vi "LVDemo1.vi"() -> ()   [LabVIEW 2010]
uses:
  toupcam.dll
  toupcam_labview.dll
panel:
  in  "Temp 3":i32
  in  "Tint 3":i32
  in  "Expotime 3":u32
  in  "ExpoGain 3":u16
  in  "Still_Width 2":i32
  in  "Still_Height 2":i32
  in  "Tab":T1(tab)
  in  "Color Default":bool
  in  "Brightness":i32(slide) scale=-64.0..64.0
  in  "Contrast":i32(slide) scale=-100.0..100.0
  in  "Gamma":i32(slide) scale=20.0..180.0
  in  "Hue":i32(slide) scale=-180.0..180.0
  in  "Saturation":i32(slide) scale=0.0..255.0
  in  "AutoExpo":bool
  in  "ExpoDefault":bool
  in  "Expotime":u32(slide) scale=294.0..2000000.0
  in  "ExpoGain":u16(slide) scale=100.0..300.0
  in  "AutoWB":bool
  in  "WBDefault":bool
  in  "Tint":i32(slide) scale=200.0..2500.0
  in  "Temp":i32(slide) scale=2000.0..15000.0
  in  "Bin/Skip Mode":bool
  in  "Chrome/Mono":bool
  in  "HFlip":bool
  in  "VFlip":bool
  in  "Frame Speed":u8(slide) scale=0.0..6.0
  out "Video":T2(plugin-control)
  in  "Cap Still Image":bool
  in  "Still Image Resolution":u16(ring) items=["2592*1944", "1280*960", "640*480"]
  in  "Cap Live Image":bool
  in  "Stop":bool
  in  "Live Resolution":u16(ring) items=["2592*1944", "1280*960", "640*480"]
  in  "?":enum32{"选项卡 1"}(tab)
  in  "Expotime_def":u32
  in  "ExpoGain_def":u16
  in  "ExpoGain_Max":u16
  in  "ExpoGain_Min":u16
  in  "Height":i32
  in  "Width":i32
  in  "Expotime_Max":u32
  in  "Expotime_Min":u32
  in  "speed":u8
  in  "height2":i32
  in  "width2":i32
  in  "Mode":bool
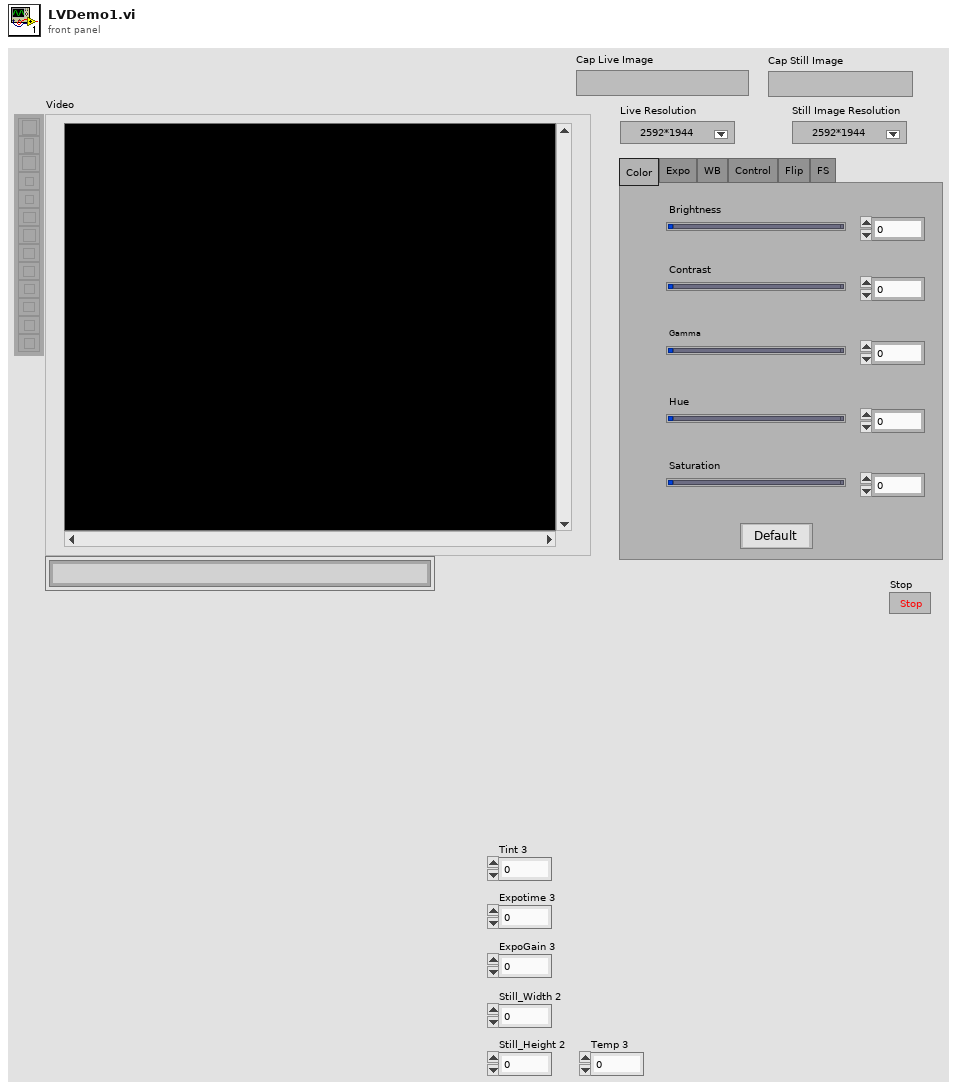
[diagram p1: front panel]
types:
  T1 = enum32{"Color", "Expo", "WB", "Control", "Flip", "FS"}
  T2 = typedef "IMAQ Image.ctl" = refnum<image>
  T3 = enum8{"Enabled", "Disabled", "Disabled and Grayed Out"}
  T4 = typedef "Image Type" = u32
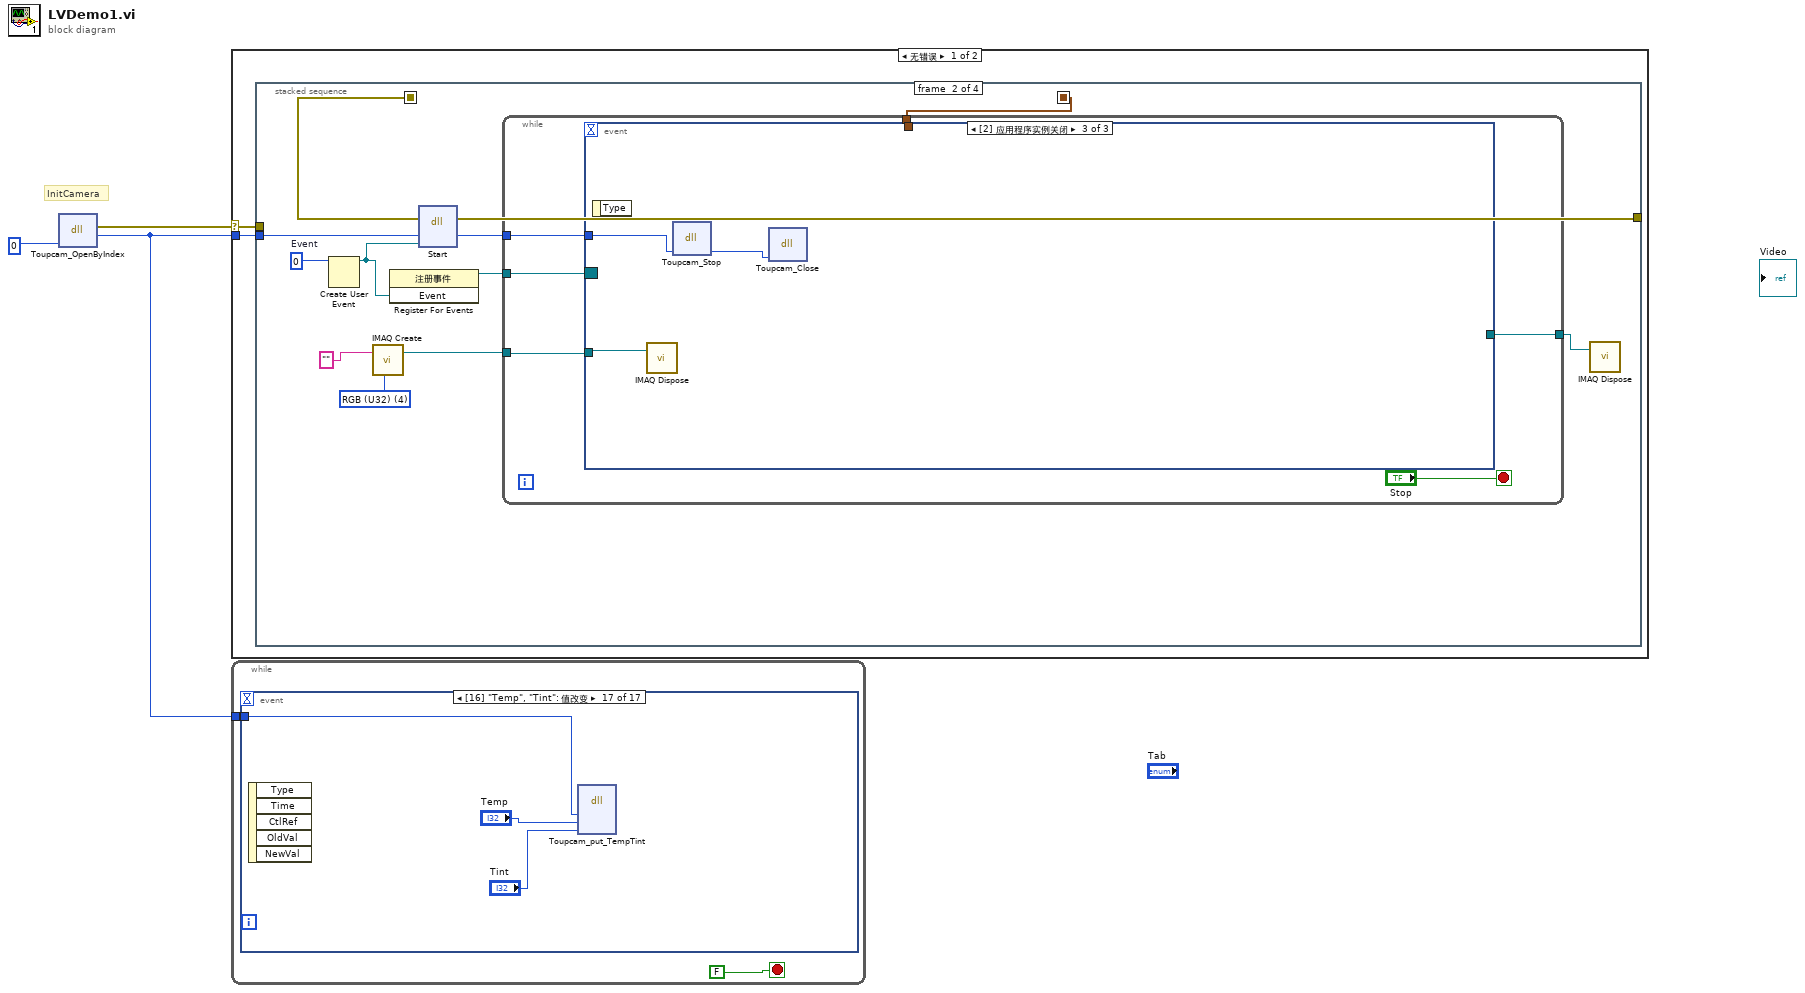
[diagram p0: block diagram]
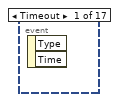
[diagram p2: hidden frame]
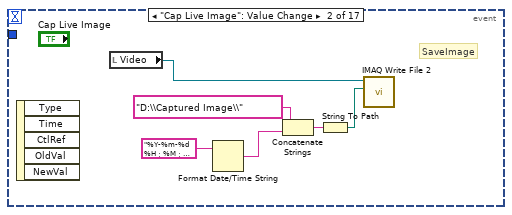
[diagram p3: hidden frame]
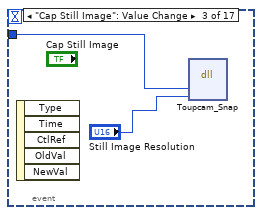
[diagram p4: hidden frame]
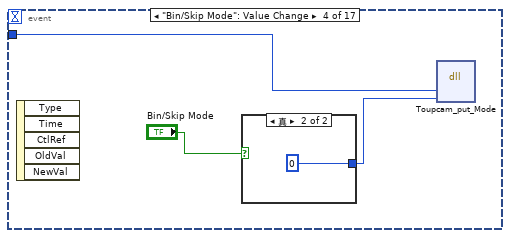
[diagram p5: hidden frame]
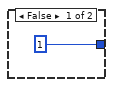
[diagram p6: hidden frame]
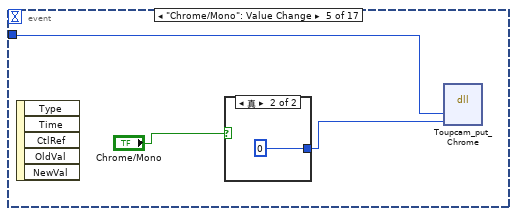
[diagram p7: hidden frame]
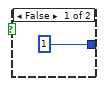
[diagram p8: hidden frame]
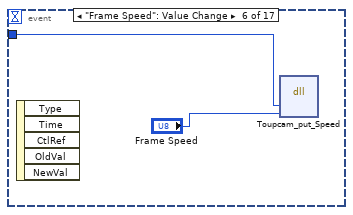
[diagram p9: hidden frame]
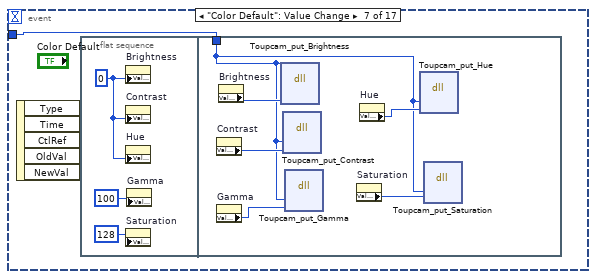
[diagram p10: hidden frame]
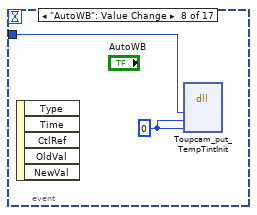
[diagram p11: hidden frame]
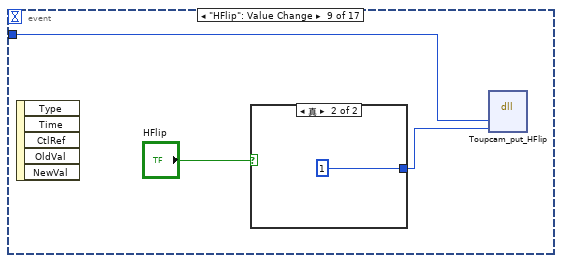
[diagram p12: hidden frame]
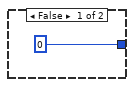
[diagram p13: hidden frame]
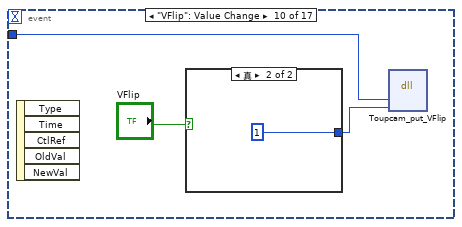
[diagram p14: hidden frame]
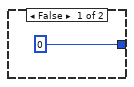
[diagram p15: hidden frame]
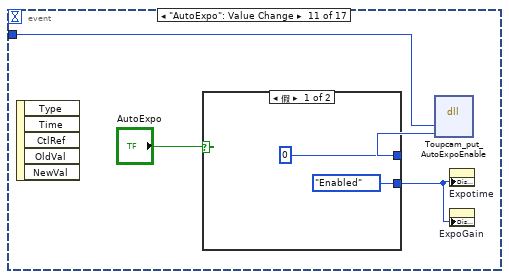
[diagram p16: hidden frame]
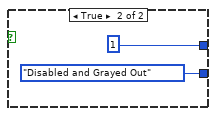
[diagram p17: hidden frame]
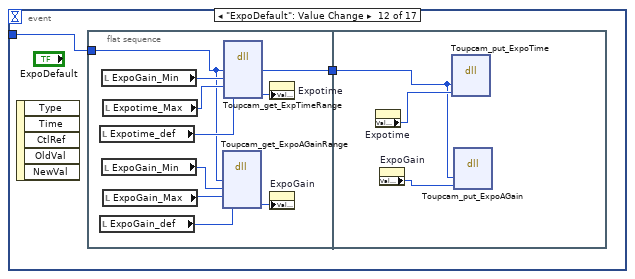
[diagram p18: hidden frame]
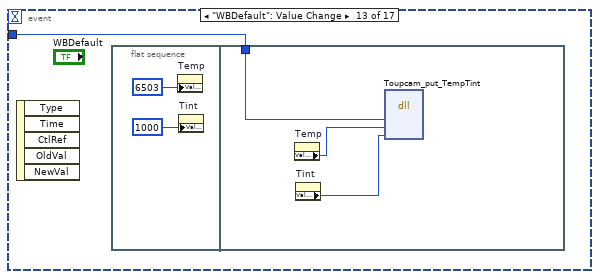
[diagram p19: hidden frame]
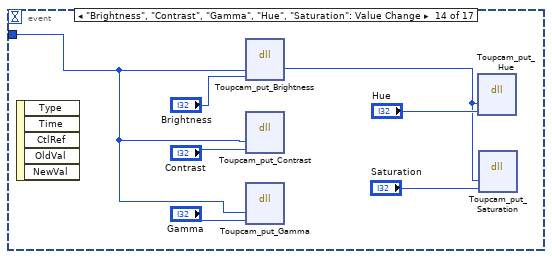
[diagram p20: hidden frame]
diagram:
  # "InitCamera"
  n1 = dll-call lib="C:/LVDemo x86/toupcam.dll" fn="Toupcam_OpenByIndex"("Index"=0) -> (error out=w3:errorcluster, "return type"=w2:i32)  [unwired: 4 in, 1 out]
  n2 = case shown="无错误" w3 {
    selector: w3 -> [w4 _]
    tunnel: w2 -> [w5 _]
    frame No Error {
      n3 = stacked-sequence {
        seq-local: [w26 _ _ _] -> [_ w72 _ _]
        seq-local: [w24 _ _ _] -> [_ w71 _ _]
        tunnel: w5 -> [w9 w69 w132 w135]
        tunnel: w4 -> [w24 _ _ w134]
        tunnel: [_ w70 _ _] -> _
        frame #0 {
          w6 = T3."Disabled and Grayed Out" ("禁用")
          w47 = 0
          # "SetSliderRange"
          # "SetCameraResolution"
          # "CameraResolution"
          # "SetSliderDefault"
          n4 = dll-call lib="C:/LVDemo x86/toupcam.dll" fn="Toupcam_put_AutoExpoEnable"("htoupcam"=w9, "bAutoExposure"=FALSE) -> ()  [unwired: 6 in, 2 out]
          n5 = dll-call lib="C:/LVDemo x86/toupcam.dll" fn="Toupcam_put_ExpoTime"("htoupcam"=w9, "Time"=5000) -> ()  [unwired: 6 in, 2 out]
          n6 = dll-call lib="C:/LVDemo x86/toupcam.dll" fn="Toupcam_get_ExpTimeRange"("htoupcam"=w9, "nMin"="Expotime_Min", "nMax"="Expotime_Max", "ndef"="Expotime_def") -> ("nMin"=w29:u32, "nMax"=w28:u32, "ndef"=w27:u32)  [unwired: 5 in, 2 out]
          n7 = dll-call lib="C:/LVDemo x86/toupcam.dll" fn="Toupcam_get_ExpoAGainRange"("htoupcam"=w9, "nmin"="ExpoGain_Min", "nmax"="ExpoGain_Max", "ndef"="ExpoGain_def") -> ("nmin"=w38:u16, "nmax"=w37:u16, "ndef"=w36:u16)  [unwired: 5 in, 2 out]
          n8 = property on="Expotime" class="Slide (strict)"("Scale.Minimum"=w29, "Scale.Maximum"=w28, "Value"=w27) -> ()  [unwired: 2 in, 2 out]
          n9 = property on="ExpoGain" class="Slide (严格)"("Scale.Minimum"=w38, "Scale.Maximum"=w37, "Value"=w36) -> ()  [unwired: 2 in, 2 out]
          n10 = dll-call lib="C:/LVDemo x86/toupcam.dll" fn="Toupcam_get_ResolutionNumber"("htoupcam"=w9) -> ("返回类型"=w15:u32, "htoupcam"=w14:i32)  [unwired: 3 in, 2 out]
          n11 = dll-call lib="C:/LVDemo x86/toupcam.dll" fn="Toupcam_get_Mode"("htoupcam"=w9, "bMode"="Mode") -> ("返回类型"=w8:i32)  [unwired: 5 in, 2 out]
          n12 = property on="Expotime" class="Slide (strict)"("DisabledEnum"=w6) -> ()  [unwired: 2 in, 2 out]
          n13 = property on="ExpoGain" class="Slide (strict)"("DisabledEnum"=w6) -> ()  [unwired: 2 in, 2 out]
          n14 = Equal To 0?(x=w8) -> (x = 0?=w7:bool)
          n15 = dll-call lib="C:/LVDemo x86/toupcam.dll" fn="Toupcam_get_MaxSpeed"("htoupcam"=w9) -> ("返回类型"=w19:u8)  [unwired: 4 in, 2 out]
          n16 = dll-call lib="C:/LVDemo x86/toupcam.dll" fn="Toupcam_get_Speed"("htoupcam"=w9, "speed"="speed") -> ("htoupcam"=w17:i32, "speed"=w20:u8)  [unwired: 4 in, 2 out]
          n17 = for {
            N: w15 -> [_]
            tunnel: w14 -> [w61]
            tunnel: [w52] -> w13 mode=indexing
            i -> [w53]
            # "Enum Res"
            n18 = dll-call lib="C:/LVDemo x86/toupcam.dll" fn="Toupcam_get_Resolution"("htoupcam"=w61, "ResNum"=w53, "pWidth"="width2", "pHeight"="height2") -> ("pWidth"=w55:i32, "pHeight"=w54:i32)  [unwired: 6 in, 2 out]
            n19 = Number To Decimal String(number=w55) -> (decimal integer string=w56:string)  [unwired: 1 in]
            n20 = Number To Decimal String(number=w54) -> (decimal integer string=w58:string)  [unwired: 1 in]
            n21 = Concatenate Strings(w56, "*", w58) -> (w52:string)
          }
          n22 = case shown="假" w7 {
            frame True {
              n23 = property on="Bin/Skip Mode" class="Bool (严格)"("DisabledEnum"=T3."Enabled" ("禁用")) -> ()  [unwired: 2 in, 2 out]
            }
            frame False {
              n24 = property on="Bin/Skip Mode" class="Bool (严格)"("DisabledEnum"=T3."Disabled and Grayed Out" ("禁用")) -> ()  [unwired: 2 in, 2 out]
            }
          }
          n25 = property on="Frame Speed" class="Slide (严格)"("Value"=w20, "Scale.Maximum"=w19, "Scale.Minimum"=0) -> ()  [unwired: 2 in, 2 out]
          n26 = dll-call lib="C:/LVDemo x86/toupcam.dll" fn="Toupcam_get_MonoMode"("htoupcam"=w17) -> ("返回类型"=w16:i32)  [unwired: 4 in, 2 out]
          n27 = case shown="0, 默认" w16 {
            frame 0, Default {
              w62 = T3."Disabled and Grayed Out" ("禁用")
              # "Mono"
              n28 = property on="Brightness" class="Slide (严格)"("DisabledEnum"=w62) -> ()  [unwired: 2 in, 2 out]
              n29 = property on="Hue" class="Slide (严格)"("DisabledEnum"=w62) -> ()  [unwired: 2 in, 2 out]
              n30 = property on="Contrast" class="Slide (严格)"("DisabledEnum"=w62) -> ()  [unwired: 2 in, 2 out]
              n31 = property on="Gamma" class="Slide (严格)"("DisabledEnum"=w62) -> ()  [unwired: 2 in, 2 out]
              n32 = property on="AutoWB" class="Bool"("DisabledEnum"=w62) -> ()  [unwired: 2 in, 2 out]
              n33 = property on="Temp" class="Slide (严格)"("DisabledEnum"=w62) -> ()  [unwired: 2 in, 2 out]
              n34 = property on="Tint" class="Slide (严格)"("DisabledEnum"=w62) -> ()  [unwired: 2 in, 2 out]
              n35 = property on="Saturation" class="Slide (严格)"("DisabledEnum"=w62) -> ()  [unwired: 2 in, 2 out]
              n36 = property on="WBDefault" class="Bool"("DisabledEnum"=w62) -> ()  [unwired: 2 in, 2 out]
              n37 = property on="Color Default" class="Bool"("DisabledEnum"=w62) -> ()  [unwired: 2 in, 2 out]
            }
            frame 1 {
              w63 = T3."Enabled" ("禁用")
              # "Mono"
              n38 = property on="Brightness" class="Slide (严格)"("DisabledEnum"=w63) -> ()  [unwired: 2 in, 2 out]
              n39 = property on="Hue" class="Slide (严格)"("DisabledEnum"=w63) -> ()  [unwired: 2 in, 2 out]
              n40 = property on="Contrast" class="Slide (严格)"("DisabledEnum"=w63) -> ()  [unwired: 2 in, 2 out]
              n41 = property on="Gamma" class="Slide (严格)"("DisabledEnum"=w63) -> ()  [unwired: 2 in, 2 out]
              n42 = property on="AutoWB" class="Bool"("DisabledEnum"=w63) -> ()  [unwired: 2 in, 2 out]
              n43 = property on="Temp" class="Slide (严格)"("DisabledEnum"=w63) -> ()  [unwired: 2 in, 2 out]
              n44 = property on="Tint" class="Slide (严格)"("DisabledEnum"=w63) -> ()  [unwired: 2 in, 2 out]
              n45 = property on="Saturation" class="Slide (严格)"("DisabledEnum"=w63) -> ()  [unwired: 2 in, 2 out]
              n46 = property on="WBDefault" class="Bool"("DisabledEnum"=w63) -> ()  [unwired: 2 in, 2 out]
              n47 = property on="Color Default" class="Bool"("DisabledEnum"=w63) -> ()  [unwired: 2 in, 2 out]
            }
          }
          n48 = dll-call lib="C:/LVDemo x86/toupcam.dll" fn="Toupcam_get_Resolution"("htoupcam"=w14, "ResNum"="Live Resolution", "pWidth"="Width", "pHeight"="Height") -> ("pWidth"=w39:i32, "pHeight"=w40:i32)  [unwired: 6 in, 2 out]
          n49 = dll-call lib="C:/LVDemo x86/toupcam.dll" fn="Toupcam_put_eSize"("htoupcam"=w14, "nResolutionIndex"="Live Resolution") -> ()  [unwired: 6 in, 2 out]
          n50 = property on="Live Resolution" class="Ring (严格)"("Strings []"=w13) -> ()  [unwired: 2 in, 2 out]
          n51 = property on="Still Image Resolution" class="Ring (严格)"("Strings []"=w13) -> ()  [unwired: 2 in, 2 out]
          n52 = Bundle("pWidth"=w39, "pHeight"=w40) -> (w26:cluster{"pWidth":i32, "pHeight":i32})  [unwired: 1 in]
          n53 = property on="Brightness" class="Slide (严格)"("Value"=w47) -> ()  [unwired: 2 in, 2 out]
          n54 = property on="Contrast" class="Slide (严格)"("Value"=w47) -> ()  [unwired: 2 in, 2 out]
          n55 = property on="Hue" class="Slide (严格)"("Value"=w47) -> ()  [unwired: 2 in, 2 out]
          n56 = property on="Gamma" class="Slide (严格)"("Value"=100) -> ()  [unwired: 2 in, 2 out]
          n57 = property on="Saturation" class="Slide (严格)"("Value"=128) -> ()  [unwired: 2 in, 2 out]
          n58 = property on="Temp" class="Slide (严格)"("Value"=6503) -> ()  [unwired: 2 in, 2 out]
          n59 = property on="Tint" class="Slide (严格)"("Value"=1000) -> ()  [unwired: 2 in, 2 out]
          n60 = property on="AutoExpo" class="Bool (严格)"("Value"=TRUE) -> ()  [unwired: 2 in, 2 out]
          n61 = property on="Bin/Skip Mode" class="Bool (严格)"("Value"=TRUE) -> ()  [unwired: 2 in, 2 out]
          n62 = property on="Chrome/Mono" class="Bool (严格)"("Value"=TRUE) -> ()  [unwired: 2 in, 2 out]
          n63 = property class="TabCtl (严格)"("Visible"=FALSE) -> ()  [unwired: 2 in, 2 out]
        }
        frame #1 {
          w68 = u32 0  # Event
          w73 = T4 4 items=["Grayscale (U8)", "Grayscale (I16)", "Grayscale (SGL)", "Complex (CSG)", "RGB (U32)", "HSL (U32)", "RGB (U64)", "Grayscale (U16)"] ("Image Type")
          n64 = Create User Event(user event datatype=w68) -> (user event=w67:refnum<user-event>)  [unwired: 1 in, 1 out]
          n65 = call "IMAQ Create"("Image Name"="", "Image Type"=w73) -> ("New Image"=w74:T2)  [unwired: 3 in, 1 out]
          n66 = register-events(w67) -> (reference out=w66:refnum<event-registration>)  [unwired: 2 in, 1 out]
          n67 = dll-call lib="C:/LVDemo x86/toupcam_labview.dll" fn="Start"(error in=w71, "htoupcam"=w69, "rwer"=w67) -> (error out=w70:errorcluster, "htoupcam"=w65:i32)  [unwired: 4 in, 1 out]
          n68 = while {
            tunnel: w74 -> [w80]
            tunnel: w72 -> [w79]
            tunnel: w66 -> [w78]
            tunnel: w65 -> [w77]
            tunnel: [w76] -> w64
            stop <- "Stop" stop-if-true
            n69 = event shown="[2] 应用程序实例关闭" {
              selector: w78 -> [_ _ _]
              dyn-events: _ -> [_ _ _]
              timeout: _ -> [_ _ _]
              tunnel: w80 -> [_ w86 w129]
              tunnel: w79 -> [_ w85 _]
              tunnel: w77 -> [_ w83 w131]
              tunnel: [_ w82 _] -> w76
              event Timeout {
                n70 = event-data() -> ()  [unwired: 1 in, 2 out]
              }
              event User Event {
                n71 = event-data() -> ("Event"=w84:u32)  [unwired: 1 in]
                n72 = case shown="5" w84 {
                  tunnel: w86 -> [w97 w105 _ _ _]
                  tunnel: w85 -> [w93 _ _ _ _]
                  tunnel: w83 -> [w89 w100 w119 w124 _]
                  tunnel: [w87 w99 _ _ _] -> w82
                  frame 4, Default {
                    # "ShowVideo"
                    n73 = Unbundle(w93) -> ("pWidth"=w91:i32, "pHeight"=w90:i32)
                    n74 = Multiply(x=w91, y=w90) -> (x*y=w95:i32)
                    n75 = Initialize Array(u32 0, w95) -> (w92:u32[])
                    n76 = dll-call lib="C:/LVDemo x86/toupcam.dll" fn="Toupcam_PullImage"("htoupcam"=w89, "pImageData"=w92, "bits"=32, "nWidth"=w91, "nHeight"=w90) -> ("pImageData"=w98:u32[])  [unwired: 8 in, 2 out]
                    n77 = Reshape Array(w98, w90, w91) -> (w96:u32[][])
                    n78 = call "IMAQ ArrayToColorImage"("Image Pixels (U32)"=w96, "Image"=w97) -> ("Image Out"=w87:T2)  [unwired: 3 in, 1 out]
                    n79 = local write "Video"(w87) -> ()
                  }
                  frame 5 {
                    # "Capture still Image"
                    n80 = property on="Still Image Resolution" class="Ring (严格)"() -> ("Value"=w101:u16)  [unwired: 2 in, 2 out]
                    n81 = dll-call lib="C:/LVDemo x86/toupcam.dll" fn="Toupcam_get_StillResolution"("htoupcam"=w100, "nIndex"=w101, "pWidth"="Still_Width 2", "pHeight"="Still_Height 2") -> ("htoupcam"=w117:i32, "pWidth"=w103:i32, "pHeight"=w104:i32)  [unwired: 5 in, 2 out]
                    n82 = Multiply(x=w103, y=w104) -> (x*y=w102:i32)
                    n83 = Initialize Array(u32 0, w102) -> (w116:u32[])
                    n84 = dll-call lib="C:/LVDemo x86/toupcam.dll" fn="Toupcam_PullStillImage"("htoupcam"=w117, "pImageData"=w116, "bits"=32, "pnWidth"=w103, "pnHeight"=w104) -> ("pImageData"=w114:u32[])  [unwired: 8 in, 2 out]
                    n85 = Reshape Array(w114, w104, w103) -> (w106:u32[][])
                    n86 = call "IMAQ ArrayToColorImage"("Image Pixels (U32)"=w106, "Image"=w105) -> ("Image Out"=w99:T2)  [unwired: 3 in, 1 out]
                    n87 = Format Date/Time String(time format string (%c)="%Y-%m-%d %H：%M：%S.bmp ") -> (date/time string=w110:string)  [unwired: 2 in]
                    n88 = Concatenate Strings("D:\\Captured Image\\", w110) -> (w107:string)
                    n89 = String To Path(string=w107) -> (path=w109:path)
                    n90 = call-poly "IMAQ Write File 2"("File Path"=w109, "Image"=w99) -> ()  [unwired: 8 in, 2 out]
                  }
                  frame 1 {
                    # "Auto Expo"
                    n91 = dll-call lib="C:/LVDemo x86/toupcam.dll" fn="Toupcam_get_ExpoAGain"("htoupcam"=w119, "ExpoGain"="ExpoGain 3") -> ("ExpoGain"=w120:u16)  [unwired: 5 in, 2 out]
                    n92 = dll-call lib="C:/LVDemo x86/toupcam.dll" fn="Toupcam_get_ExpoTime"("htoupcam"=w119, "Expotime"="Expotime 3") -> ("Expotime"=w121:u32)  [unwired: 5 in, 2 out]
                    n93 = property on="ExpoGain" class="Slide (严格)"("Value"=w120) -> ()  [unwired: 2 in, 2 out]
                    n94 = property on="Expotime" class="Slide (严格)"("Value"=w121) -> ()  [unwired: 2 in, 2 out]
                  }
                  frame 2 {
                    # "Auto WhiteBalance"
                    n95 = dll-call lib="C:/LVDemo x86/toupcam.dll" fn="Toupcam_get_TempTint"("htoupcam"=w124, "Temp"="Temp 3", "Tint"="Tint 3") -> ("Temp"=w126:i32, "Tint"=w125:i32)  [unwired: 5 in, 2 out]
                    n96 = property on="Tint" class="Slide (严格)"("Value"=w125) -> ()  [unwired: 2 in, 2 out]
                    n97 = property on="Temp" class="Slide (严格)"("Value"=w126) -> ()  [unwired: 2 in, 2 out]
                  }
                  frame 3 {
                  }
                }
              }
              event Application Instance Close {
                n98 = event-data() -> ()  [unwired: 1 in, 1 out]
                n99 = call "IMAQ Dispose"("Image"=w129) -> ()  [unwired: 5 in, 1 out]
                n100 = dll-call lib="C:/LVDemo x86/toupcam.dll" fn="Toupcam_Stop"("htoupcam"=w131) -> ("htoupcam"=w130:i32)  [unwired: 4 in, 2 out]
                n101 = dll-call lib="C:/LVDemo x86/toupcam.dll" fn="Toupcam_Close"("htoupcam"=w130) -> ()  [unwired: 5 in, 2 out]
              }
            }
          }
          n102 = call "IMAQ Dispose"("Image"=w64) -> ()  [unwired: 5 in, 1 out]
        }
        frame #2 {
          n103 = dll-call lib="C:/LVDemo x86/toupcam.dll" fn="Toupcam_Stop"("htoupcam"=w132) -> ()  [unwired: 5 in, 2 out]
        }
        frame #3 {
          n104 = dll-call lib="C:/LVDemo x86/toupcam.dll" fn="Toupcam_Close"(error in=w134, "htoupcam"=w135) -> ()  [unwired: 4 in, 2 out]
          n105 = Stop(stop? (T)=TRUE) -> ()
        }
      }
    }
    frame Error {
    }
  }
  n106 = while {
    tunnel: w2 -> [w136]
    stop <- FALSE ("停止 2") stop-if-true
    n107 = event shown="[16] \"Temp\", \"Tint\": 值改变" {
      selector: _ -> [_ _ _ _ _ _ _ _ _ _ _ _ _ _ _ _ _]
      dyn-events: _ -> [_ _ _ _ _ _ _ _ _ _ _ _ _ _ _ _ _]
      timeout: _ -> [_ _ _ _ _ _ _ _ _ _ _ _ _ _ _ _ _]
      tunnel: w136 -> [_ _ w145 w148 w153 w156 w158 w169 w172 w177 w183 w189 w203 w210 w216 w218 w222]
      event Timeout {
        n108 = event-data() -> ()  [unwired: 1 in, 2 out]
      }
      event "Cap Live Image": Value Change {
        # "SaveImage"
        n109 = event-data() -> ()  [unwired: 1 in, 5 out]
        n110 = local read "Video"() -> (w138:T2)
        n111 = Format Date/Time String(time format string (%c)="%Y-%m-%d %H：%M：%S.bmp ") -> (date/time string=w142:string)  [unwired: 2 in]
        n112 = Concatenate Strings("D:\\Captured Image\\", w142) -> (w139:string)
        n113 = String To Path(string=w139) -> (path=w141:path)
        n114 = call-poly "IMAQ Write File 2"("File Path"=w141, "Image"=w138) -> ()  [unwired: 8 in, 2 out]
      }
      event "Cap Still Image": Value Change {
        n115 = event-data() -> ()  [unwired: 1 in, 5 out]
        n116 = dll-call lib="C:/LVDemo x86/toupcam.dll" fn="Toupcam_Snap"("htoupcam"=w145, "ResIndex"="Still Image Resolution") -> ()  [unwired: 6 in, 2 out]
      }
      event "Bin/Skip Mode": Value Change {
        n117 = event-data() -> ()  [unwired: 1 in, 5 out]
        n118 = case shown="真" "Bin/Skip Mode" {
          tunnel: [1 0] -> w146
          frame False {
          }
          frame True {
          }
        }
        n119 = dll-call lib="C:/LVDemo x86/toupcam.dll" fn="Toupcam_put_Mode"("htoupcam"=w148, "mode"=w146) -> ()  [unwired: 6 in, 2 out]
      }
      event "Chrome/Mono": Value Change {
        n120 = event-data() -> ()  [unwired: 1 in, 5 out]
        n121 = case shown="真" "Chrome/Mono" {
          tunnel: [1 0] -> w151
          frame False {
          }
          frame True {
          }
        }
        n122 = dll-call lib="C:/LVDemo x86/toupcam.dll" fn="Toupcam_put_Chrome"("htoupcam"=w153, "chrome"=w151) -> ()  [unwired: 6 in, 2 out]
      }
      event "Frame Speed": Value Change {
        n123 = event-data() -> ()  [unwired: 1 in, 5 out]
        n124 = dll-call lib="C:/LVDemo x86/toupcam.dll" fn="Toupcam_put_Speed"("htoupcam"=w156, "Speed"="Frame Speed") -> ()  [unwired: 6 in, 2 out]
      }
      event "Color Default": Value Change {
        n125 = event-data() -> ()  [unwired: 1 in, 5 out]
        n126 = flat-sequence {
          tunnel: w158 -> [w162]
          frame #0 {
            w161 = 0
            n127 = property on="Brightness" class="Slide (严格)"("Value"=w161) -> ()  [unwired: 2 in, 2 out]
            n128 = property on="Contrast" class="Slide (严格)"("Value"=w161) -> ()  [unwired: 2 in, 2 out]
            n129 = property on="Hue" class="Slide (严格)"("Value"=w161) -> ()  [unwired: 2 in, 2 out]
            n130 = property on="Saturation" class="Slide (严格)"("Value"=128) -> ()  [unwired: 2 in, 2 out]
            n131 = property on="Gamma" class="Slide (严格)"("Value"=100) -> ()  [unwired: 2 in, 2 out]
          }
          frame #1 {
            n132 = property on="Contrast" class="Slide (严格)"() -> ("Value"=w166:i32)  [unwired: 2 in, 2 out]
            n133 = property on="Gamma" class="Slide (严格)"() -> ("Value"=w165:i32)  [unwired: 2 in, 2 out]
            n134 = property on="Brightness" class="Slide (严格)"() -> ("Value"=w167:i32)  [unwired: 2 in, 2 out]
            n135 = dll-call lib="C:/LVDemo x86/toupcam.dll" fn="Toupcam_put_Brightness"("htoupcam"=w162, "Brightness"=w167) -> ()  [unwired: 6 in, 2 out]
            n136 = dll-call lib="C:/LVDemo x86/toupcam.dll" fn="Toupcam_put_Contrast"("htoupcam"=w162, "Contrast"=w166) -> ()  [unwired: 6 in, 2 out]
            n137 = dll-call lib="C:/LVDemo x86/toupcam.dll" fn="Toupcam_put_Gamma"("htoupcam"=w162, "Gamma"=w165) -> ()  [unwired: 6 in, 2 out]
            n138 = property on="Saturation" class="Slide (严格)"() -> ("Value"=w163:i32)  [unwired: 2 in, 2 out]
            n139 = property on="Hue" class="Slide (严格)"() -> ("Value"=w164:i32)  [unwired: 2 in, 2 out]
            n140 = dll-call lib="C:/LVDemo x86/toupcam.dll" fn="Toupcam_put_Hue"("htoupcam"=w162, "Hue"=w164) -> ()  [unwired: 6 in, 2 out]
            n141 = dll-call lib="C:/LVDemo x86/toupcam.dll" fn="Toupcam_put_Saturation"("htoupcam"=w162, "Saturation"=w163) -> ()  [unwired: 6 in, 2 out]
          }
        }
      }
      event "AutoWB": Value Change {
        w168 = 0
        n142 = event-data() -> ()  [unwired: 1 in, 5 out]
        n143 = dll-call lib="C:/LVDemo x86/toupcam.dll" fn="Toupcam_put_TempTintInit"("htoupcam"=w169, "fnTTProc"=w168, "pTTCtx"=w168) -> ()  [unwired: 7 in, 2 out]
      }
      event "HFlip": Value Change {
        n144 = event-data() -> ()  [unwired: 1 in, 5 out]
        n145 = case shown="真" "HFlip" {
          tunnel: [0 1] -> w170
          frame False {
          }
          frame True {
          }
        }
        n146 = dll-call lib="C:/LVDemo x86/toupcam.dll" fn="Toupcam_put_HFlip"("htoupcam"=w172, "bHFlip"=w170) -> ()  [unwired: 6 in, 2 out]
      }
      event "VFlip": Value Change {
        n147 = event-data() -> ()  [unwired: 1 in, 5 out]
        n148 = case shown="真" "VFlip" {
          tunnel: [0 1] -> w175
          frame False {
          }
          frame True {
          }
        }
        n149 = dll-call lib="C:/LVDemo x86/toupcam.dll" fn="Toupcam_put_VFlip"("htoupcam"=w177, "bVFlip"=w175) -> ()  [unwired: 6 in, 2 out]
      }
      event "AutoExpo": Value Change {
        n150 = event-data() -> ()  [unwired: 1 in, 5 out]
        n151 = case shown="假" "AutoExpo" {
          tunnel: [0 1] -> w180
          tunnel: [T3."Enabled" ("禁用") T3."Disabled and Grayed Out" ("禁用")] -> w181
          frame False {
          }
          frame True {
          }
        }
        n152 = dll-call lib="C:/LVDemo x86/toupcam.dll" fn="Toupcam_put_AutoExpoEnable"("HToupcam"=w183, "bAutoExposure"=w180) -> ()  [unwired: 6 in, 2 out]
        n153 = property on="Expotime" class="Slide (严格)"("DisabledEnum"=w181) -> ()  [unwired: 2 in, 2 out]
        n154 = property on="ExpoGain" class="Slide (严格)"("DisabledEnum"=w181) -> ()  [unwired: 2 in, 2 out]
      }
      event "ExpoDefault": Value Change {
        n155 = event-data() -> ()  [unwired: 1 in, 5 out]
        n156 = flat-sequence {
          tunnel: w189 -> [w191]
          tunnel: [w190] -> w188
          tunnel: w188 -> [w200]
          frame #0 {
            n157 = local read "Expotime_def"() -> (w197:u32)
            n158 = local read "ExpoGain_def"() -> (w193:u16)
            n159 = local read "ExpoGain_Min"() -> (w199:u16)
            n160 = local read "ExpoGain_Min"() -> (w195:u16)
            n161 = local read "Expotime_Max"() -> (w198:u32)
            n162 = local read "ExpoGain_Max"() -> (w194:u16)
            n163 = dll-call lib="C:/LVDemo x86/toupcam.dll" fn="Toupcam_get_ExpoAGainRange"("htoupcam"=w191, "min"=w195, "max"=w194, "def"=w193) -> ("def"=w196:u16)  [unwired: 7 in, 2 out]
            n164 = dll-call lib="C:/LVDemo x86/toupcam.dll" fn="Toupcam_get_ExpTimeRange"("htoupcam"=w191, "Min"=w199, "Max"=w198, "def"=w197) -> ("htoupcam"=w190:i32, "def"=w192:u32)  [unwired: 6 in, 2 out]
            n165 = property on="Expotime" class="Slide (严格)"("Value"=w192) -> ()  [unwired: 2 in, 2 out]
            n166 = property on="ExpoGain" class="Slide (严格)"("Value"=w196) -> ()  [unwired: 2 in, 2 out]
          }
          frame #1 {
            n167 = property on="Expotime" class="Slide (严格)"() -> ("Value"=w202:u32)  [unwired: 2 in, 2 out]
            n168 = property on="ExpoGain" class="Slide (严格)"() -> ("Value"=w201:u16)  [unwired: 2 in, 2 out]
            n169 = dll-call lib="C:/LVDemo x86/toupcam.dll" fn="Toupcam_put_ExpoTime"("htoupcam"=w200, "Expotime"=w202) -> ()  [unwired: 6 in, 2 out]
            n170 = dll-call lib="C:/LVDemo x86/toupcam.dll" fn="Toupcam_put_ExpoAGain"("htoupcam"=w200, "ExpoGain"=w201) -> ()  [unwired: 6 in, 2 out]
          }
        }
      }
      event "WBDefault": Value Change {
        n171 = event-data() -> ()  [unwired: 1 in, 5 out]
        n172 = flat-sequence {
          tunnel: w203 -> [w208]
          frame #0 {
            n173 = property on="Temp" class="Slide (严格)"("Value"=6503) -> ()  [unwired: 2 in, 2 out]
            n174 = property on="Tint" class="Slide (严格)"("Value"=1000) -> ()  [unwired: 2 in, 2 out]
          }
          frame #1 {
            n175 = property on="Temp" class="Slide (严格)"() -> ("Value"=w207:i32)  [unwired: 2 in, 2 out]
            n176 = property on="Tint" class="Slide (严格)"() -> ("Value"=w206:i32)  [unwired: 2 in, 2 out]
            n177 = dll-call lib="C:/LVDemo x86/toupcam.dll" fn="Toupcam_put_TempTint"("htoupcam"=w208, "Temp"=w207, "Tint"=w206) -> ()  [unwired: 7 in, 2 out]
          }
        }
      }
      event "Brightness", "Contrast", "Gamma", "Hue", "Saturation": Value Change {
        n178 = event-data() -> ()  [unwired: 1 in, 5 out]
        n179 = dll-call lib="C:/LVDemo x86/toupcam.dll" fn="Toupcam_put_Brightness"("htoupcam"=w210, "Brightness"="Brightness") -> ("htoupcam"=w209:i32)  [unwired: 5 in, 2 out]
        n180 = dll-call lib="C:/LVDemo x86/toupcam.dll" fn="Toupcam_put_Contrast"("htoupcam"=w210, "Contrast"="Contrast") -> ()  [unwired: 6 in, 2 out]
        n181 = dll-call lib="C:/LVDemo x86/toupcam.dll" fn="Toupcam_put_Gamma"("htoupcam"=w210, "Gamma"="Gamma") -> ()  [unwired: 6 in, 2 out]
        n182 = dll-call lib="C:/LVDemo x86/toupcam.dll" fn="Toupcam_put_Hue"("htoupcam"=w209, "Hue"="Hue") -> ()  [unwired: 6 in, 2 out]
        n183 = dll-call lib="C:/LVDemo x86/toupcam.dll" fn="Toupcam_put_Saturation"("htoupcam"=w209, "Saturation"="Saturation") -> ()  [unwired: 6 in, 2 out]
      }
      event "Expotime": Value Change {
        n184 = event-data() -> ()  [unwired: 1 in, 5 out]
        n185 = dll-call lib="C:/LVDemo x86/toupcam.dll" fn="Toupcam_put_ExpoTime"("htoupcam"=w216, "Expotime"="Expotime") -> ()  [unwired: 6 in, 2 out]
      }
      event "ExpoGain": Value Change {
        n186 = event-data() -> ()  [unwired: 1 in, 5 out]
        n187 = dll-call lib="C:/LVDemo x86/toupcam.dll" fn="Toupcam_put_ExpoAGain"("htoupcam"=w218, "ExpoGain"="ExpoGain") -> ()  [unwired: 6 in, 2 out]
      }
      event "Temp", "Tint": Value Change {
        n188 = event-data() -> ()  [unwired: 1 in, 5 out]
        n189 = dll-call lib="C:/LVDemo x86/toupcam.dll" fn="Toupcam_put_TempTint"("htoupcam"=w222, "Temp"="Temp", "Tint"="Tint") -> ()  [unwired: 7 in, 2 out]
      }
    }
  }
